vi "Turret Controller.vi"(8 "error in":errorcluster) -> ()   [LabVIEW 2019]
doc: "This VI executes continuously carrying out the current operation and responding to updates or new operations. It will often contain the timing or control code that is difficult to place directly in TeleOp. This VI generally opens all sensors and motors and isolates the rest of the robot code from knowing how the operations are carried out."
uses:
  <vilib>/Rock Robotics/WPI/Framework/Completion Status.ctl
  Turret Setpoints.ctl
  Turret Operations.ctl
  <vilib>/Rock Robotics/Network Tables/NT Write Boolean.vi
panel:
  in  "Tab Control":T1(tab)
  in  "Buttons":cluster{"Execute Cmd":bool, "Abort Cmd":bool}
  out "Command Timing":cluster{"Start Time (ms)":u32, "Iterations":i32}
  out "Status":T2
  in  "Interactive Values":T3
  in  "PIDF gains":cluster{"Kp":dbl, "Ki":dbl, "Kd":dbl, "Kf":dbl}={"Kp"=0.06, "Ki"=0.0, "Kd"=0.0, "Kf"=0.0} {"Kf" format="%.3f"; "Kd" format="%.3f"; "Ki" format="%.3f"; "Kp" format="%.3f"}
  in  "i Zone":dbl format="%.2f"
  out "Left and Right Motor Values":T5(graph)
  in  "output range in":cluster{"output high":dbl, "output low":dbl}={"output high"=0.6, "output low"=-0.6} {"output low" format="%.2f"; "output high" format="%.2f"}
  in  "Allowed Error":dbl
  out "Process Variable Vs. Setpoint":cluster{dbl, "setpoint":dbl}(graph)
  out "Current\nCmd":string
  # "Tip: It may be helpful to observe inputs and sensor values.\nYou may also want to display tuning or debugging controls."
  # "Interactive Command: You may fill in the settings for a command\nand schedule it with the Execute button. You can observe and abort\nany command while fine tuning the code for the controller."
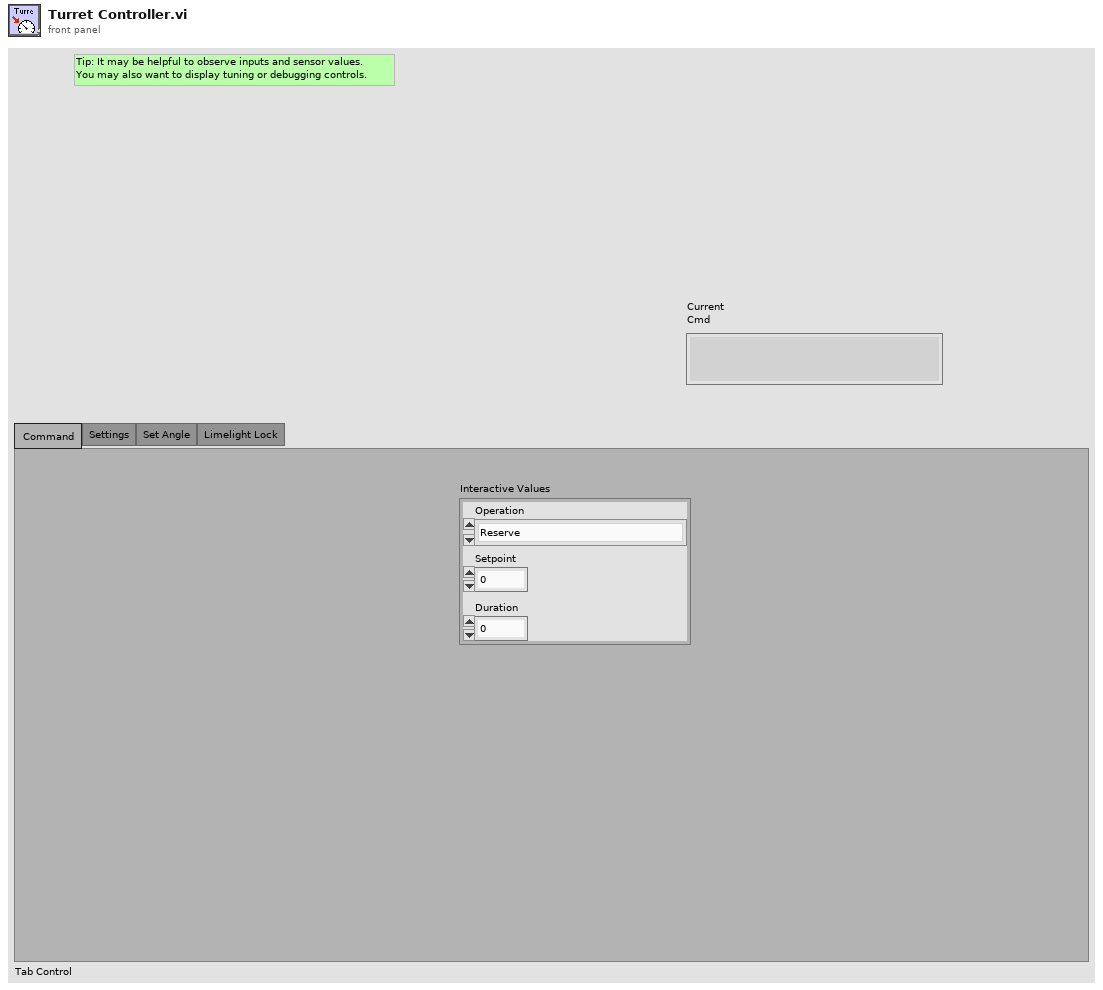
[diagram p1: front panel]
types:
  T1 = enum32{"Command ", "Settings", "Set Angle", "Limelight Lock"}
  T2 = typedef "Completion Status.ctl" = enum16{"Successful", "Aborted", "Incomplete"}
  T3 = typedef "Turret Setpoints.ctl" = cluster{"Operation":T4, "Setpoint":dbl, "Duration":dbl}
  T4 = typedef "Turret Operations.ctl" = enum16{"Reserve", "Read Current", "Immediate", "Set Angle", "Limelight Lock"}
  T5 = cluster{"Left Motor Value":dbl, "Right Motor Value":dbl}
  T6 = typedef "Command Status Info.ctl" = cluster{"Name":string, "Status":T2, "notifier out":T7}
  T7 = typedef "Completion Notifier.ctl" = refnum<notifier>
  T8 = cluster{"Current Command":T3, "Command Timing":cluster{"Start Time (ms)":u32, "Iterations":i32}, "Command Arguments":cluster{"Command Info":T6, "Description":string, "Default Command":T3, "queue out":refnum<queue>, "Subsystem Name":string}}
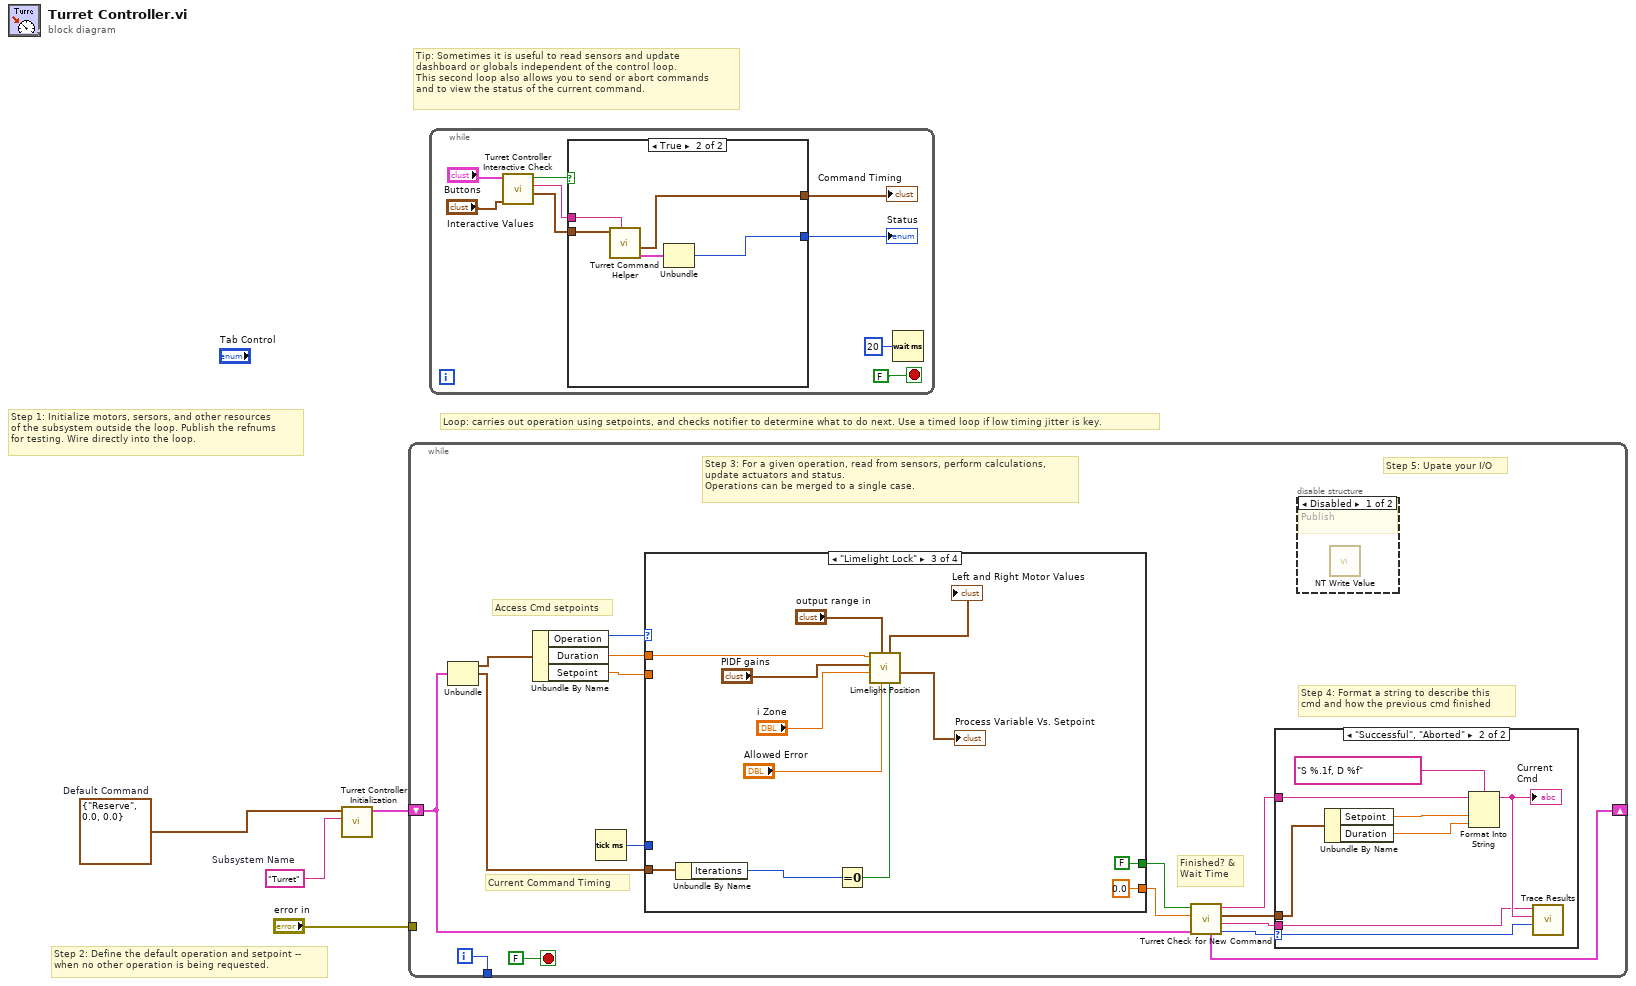
[diagram p0: block diagram]
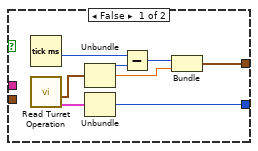
[diagram p2: hidden frame]
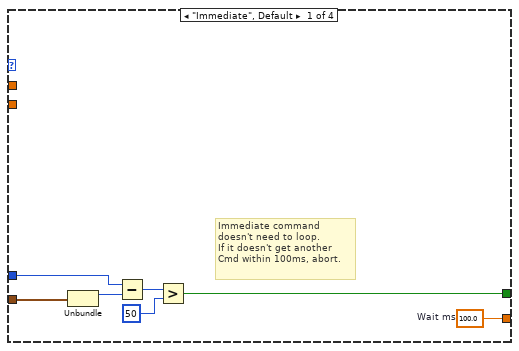
[diagram p5: hidden frame]
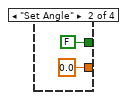
[diagram p6: hidden frame]
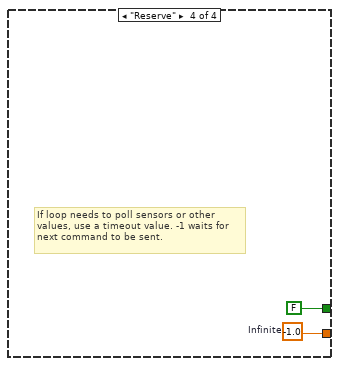
[diagram p7: hidden frame]
diagram:
  w1 = T3 {"Operation"=enum."Reserve", "Setpoint"=0.0, "Duration"=0.0}  # Default Command
  w2 = "Turret"  # Subsystem Name
  # "Tip: Sometimes it is useful to read sensors and update\ndashboard or globals independent of the control loop.\nThis second loop also allows you to send or abort commands\nand to view the status of the current command."
  # "Step 2: Define the default operation and setpoint --\nwhen no other operation is being requested."
  # "Step 1: Initialize motors, sersors, and other resources\nof the subsystem outside the loop. Publish the refnums\nfor testing. Wire directly into the loop."
  # "Loop: carries out operation using setpoints, and checks notifier to determine what to do next. Use a timed loop if low timing jitter is key."
  n1 = call "Turret Controller Initialization.vi"("Subsystem Name"=w2, "Default Command"=w1) -> ("Current Command"=w3:T8)  [unwired: 9 in]
  n2 = while {
    shift-right: [w12] -> _
    shift-left: w3 -> [w5]
    tunnel: [w19] -> _
    tunnel: "error in" -> [_]
    i -> [w19]
    stop <- FALSE stop-if-true
    # "Step 5: Upate your I/O"
    # "Step 4: Format a string to describe this\ncmd and how the previous cmd finished"
    # "Current Command Timing"
    # "Access Cmd setpoints"
    # "Finished? &\nWait Time"
    # "Step 3: For a given operation, read from sensors, perform calculations,\nupdate actuators and status.\nOperations can be merged to a single case."
    n3 = Unbundle(w5) -> ("Current Command"=w18:T3, "Command Timing"=w14:cluster{"Start Time (ms)":u32, "Iterations":i32})  [unwired: 1 out]
    n4 = Unbundle By Name(w18) -> ("Operation"=w17:T4, "Duration"=w16:dbl, "Setpoint"=w13:dbl)
    n5 = Tick Count (ms)() -> (millisecond timer value=w15:u32)
    n6 = case shown="\"Limelight Lock\"" w17 {
      tunnel: [w35 0.0 ("Infinite") 0.0 ("Infinite") w51] -> w10
      tunnel: [w29 FALSE ("ignore previous (F)") FALSE ("ignore previous (F)") FALSE ("ignore previous (F)")] -> w11
      tunnel: w14 -> [w31 _ w41 _]
      tunnel: w16 -> [_ _ w49 _]
      tunnel: w15 -> [w30 _ _ _]
      tunnel: w13 -> [_ _ _ _]
      frame "Immediate", Default {
        w35 = 100.0  # Wait ms
        # "Immediate command\ndoesn't need to loop.\nIf it doesn't get another\nCmd within 100ms, abort."
        n7 = Unbundle(w31) -> ("Start Time (ms)"=w34:u32)  [unwired: 1 out]
        n8 = Subtract(x=w30, y=w34) -> (x-y=w33:u32)
        n9 = Greater?(x=w33, y=u8 50 ("Left Motor")) -> (0:w29:bool)
      }
      frame "Set Angle" {
      }
      frame "Limelight Lock" {
        n10 = Unbundle By Name(w41) -> ("Iterations"=w42:i32)
        n11 = Equal To 0?(x=w42) -> (x = 0?=w40:bool)
        n12 = call "Limelight Position.vi"("Boolean"=w40, "Allowed Error"="Allowed Error", "output range in"="output range in", "i Zone"="i Zone", "PIDF gains"="PIDF gains", "Left Setpoint"=w49) -> ("Process Variable Vs. Setpoint"=→"Process Variable Vs. Setpoint":cluster{dbl, "setpoint":dbl}, "Left and Right Motor Values"=→"Left and Right Motor Values":T5)  [unwired: 2 in, 2 out]
      }
      frame "Reserve" {
        w51 = -1.0  # Infinite
        # "If loop needs to poll sensors or other\nvalues, use a timeout value. -1 waits for\nnext command to be sent."
      }
    }
    n13 = call "Turret Check for New Command.vi"("Current Command"=w5, "Wait time (ms)"=w10, "Finished?"=w11) -> ("Completion"=w6:T2, "Subsystem Name"=w7:string, "Current Command"=w8:T3, "Initial Trace String"=w9:string, "NextCommand"=w12:T8)  [unwired: 4 in]
    n14 = case shown="\"Successful\", \"Aborted\"" w6 {
      selector: w6 -> [_ w28]
      tunnel: w9 -> [_ w24]
      tunnel: w8 -> [_ w25]
      tunnel: w7 -> [_ w21]
      frame "Incomplete", Default {
        # "Continuing current command"
      }
      frame "Successful", "Aborted" {
        # "Report and setup for next command"
        n15 = Unbundle By Name(w25) -> ("Setpoint"=w27:dbl, "Duration"=w22:dbl)
        n16 = Format Into String(format string="S %.1f, D %f", initial string=w24, w27, w22) -> (resulting string=w23:string)  [unwired: 1 in, 1 out]
        "Current\nCmd" <- w23
        n17 = call <vilib>:"Trace Results.vi"("Status of previous command"=w28, "Description"=w23, "Subsystem"=w21) -> ()  [unwired: 9 in]
      }
    }
    n18 = disable-structure shown="Disabled" {
      frame Disabled {
        # "Publish"
        n19 = call-poly <vilib>:"NT Write Value.vi"() -> ()  [unwired: 11 in, 1 out]
      }
      frame Enabled {
      }
    }
  }
  n20 = while {
    stop <- FALSE stop-if-true
    n21 = call "Turret Controller Interactive Check.vi"("Interactive Command in"="Interactive Values", "Buttons"="Buttons") -> ("Interactive Command out"=w55:T3, "Trace String"=w56:string, "Schedule"=w57:bool)  [unwired: 7 in]
    n22 = case shown="True" w57 {
      tunnel: [w68 w73] -> w54
      tunnel: w55 -> [_ w71]
      tunnel: [w64 w69] -> w53
      tunnel: w56 -> [_ w72]
      frame False {
        n23 = Tick Count (ms)() -> (millisecond timer value=w63:u32)
        n24 = call "Read Turret Operation.vi"() -> ("Command Info"=w61:T6, "SubSystem Data"=w62:T3)  [unwired: 9 in, 1 out]
        n25 = Unbundle(w62) -> ("Operation"=w67:T4, "Setpoint"=w65:dbl)  [unwired: 1 out]
        n26 = Unbundle(w61) -> ("Status"=w68:T2)  [unwired: 2 out]
        n27 = Subtract(x=w63, y=w67) -> (x-y=w66:u32)
        n28 = Bundle(w66, "Setpoint"=w65) -> (w64:cluster{u32, "Setpoint":dbl})  [unwired: 1 in]
      }
      frame True {
        n29 = call "Turret Command Helper.vi"("Description"=w72, "SubSystem Data"=w71) -> ("Command Info Out"=w70:T6, "Command Timing"=w69:cluster{"Start Time (ms)":u32, "Iterations":i32})  [unwired: 7 in, 1 out]
        n30 = Unbundle(w70) -> ("Status"=w73:T2)  [unwired: 2 out]
      }
    }
    "Status" <- w54
    "Command Timing" <- w53
    n31 = Wait (ms)(milliseconds to wait=u32 20) -> ()  [unwired: 1 out]
  }
